vi "mean12.vi"(2 "Y":dbl[](array[numeric])) -> (6 "mean":dbl, 7 "dY":dbl caption="Шаг\nквантования\nпо уровню", 8 "std":dbl)   [LabVIEW 2010]
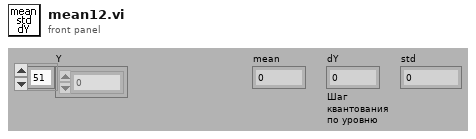
[diagram p1: front panel]
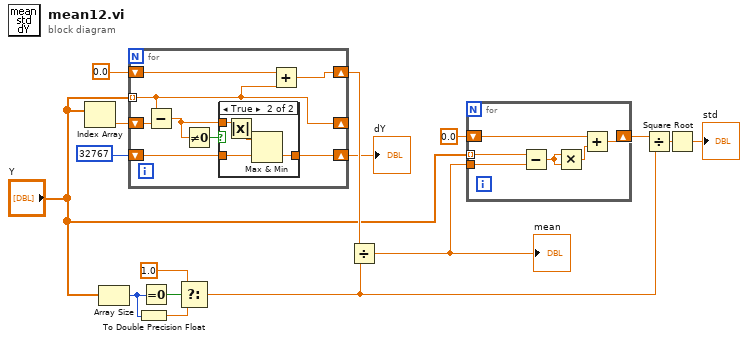
[diagram p0: block diagram]
diagram:
  n1 = Index Array(array="Y") -> (element=w9:dbl)  [unwired: 1 in]
  n2 = Array Size(array="Y") -> (size(s)=w11:i32)
  n3 = for {
    shift-right: [w17] -> _
    shift-left: w9 -> [w24]
    tunnel: "Y" -> [w17] mode=indexing
    shift-right: [w21] -> w10
    shift-left: i16 32767 ("max(x,y)") -> [w20]
    shift-right: [w19] -> w16
    shift-left: 0.0 -> [w18]
    n4 = Subtract(x=w17, y=w24) -> (x-y=w23:dbl)
    n5 = Not Equal To 0?(x=w23) -> (x != 0?=w22:bool)
    n6 = case shown="True" w22 {
      tunnel: w23 -> [_ w28]
      tunnel: [w25 w27] -> w21
      tunnel: w20 -> [w25 w26]
      frame False {
      }
      frame True {
        n7 = Absolute Value(x=w28) -> (abs(x)=w29:dbl)
        n8 = Max & Min(x=w29, y=w26) -> (min(x,y)=w27:dbl)  [unwired: 1 out]
      }
    }
    n9 = Add(x=w18, y=w17) -> (x+y=w19:dbl)
  }
  "dY" <- w10
  n10 = To Double Precision Float(number=w11) -> (double precision float=w13:dbl)
  n11 = Equal To 0?(x=w11) -> (x = 0?=w12:bool)
  n12 = Select(t=1.0, s=w12, f=w13) -> (s? t:f=w1:dbl)
  n13 = Divide(x=w16, y=w1) -> (x/y=w3:dbl)
  "mean" <- w3
  n14 = for {
    tunnel: "Y" -> [w30] mode=indexing
    tunnel: w3 -> [w35]
    shift-right: [w32] -> w7
    shift-left: 0.0 -> [w31]
    n15 = Subtract(x=w30, y=w35) -> (x-y=w34:dbl)
    n16 = Multiply(x=w34, y=w34) -> (x*y=w33:dbl)
    n17 = Add(x=w31, y=w33) -> (x+y=w32:dbl)
  }
  n18 = Divide(x=w7, y=w1) -> (x/y=w6:dbl)
  n19 = Square Root(x=w6) -> (sqrt(x)=→"std":dbl)
